vi "Ch_setup_string.vi"(6 "Ch & spans":T1[](array[typedef]) {"Sync Delay (ms)" format="%.3f"}) -> (1 "Output string":string)   [LabVIEW 2017]
uses:
  Controls/Ch_and_Spans.ctl
  Globals/Meas_global.vi
panel:
  out "length":i32
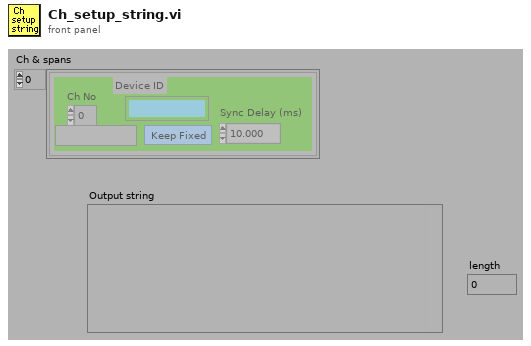
[diagram p1: front panel]
types:
  T1 = typedef "Ch_and_Spans.ctl" = cluster{"Sync Delay (ms)":dbl, "Ch No":i16, "Var name":string, "Use Latest Calib":bool, "Device ID":string}
  T2 = typedef "Analysis_info_cluster.ctl" = cluster{"Colour":u32, "Inst type":T3, "Inst name":string, "Symbol":string, "Code name":string, "Extra Info":string, "Inst Array":T4, "Extra Titles":string[], "Extra Values":string[], "U":dbl, "u^2":dbl, "u^3":dbl, "u^4":dbl, "Skew_u":dbl, "Kurt_u":dbl, "Sd Error in Mean":dbl, "% u'/U":dbl, "X":dbl, "Y":dbl, "Z":dbl, "Timescale integral Estimate":dbl, "Sd Error in Variance":dbl, "Calib File":path, "Calib Constants":dbl[], "Output Position":bool, "Full Stats":bool, "Av Sampling Rate":dbl, "Av No of Samples":dbl, "Total Meas Time (s)":dbl, "ADAM Ch Name":string, "Max value":dbl, "Min value":dbl, "Sync Delay Time (s)":dbl, "Device ID":string}
  T3 = typedef "Inst_type.ctl" = enum16{"Propeller anemometer", "Raw voltage", "Pressure Transducer", "Pitot-static tube", "Preston tube", "Hot wire", "Cross wire 1", "Cross wire 2", "Generic Linear", "Generic Polynomial", "Generic BackPoly", "Fast FID", "Thermocouple", "Cold wire", "Pulsed Wire", "LDA Vel", "LDA Tran time", "LDA Arr time", "Microphone"}
  T4 = typedef "Instrument_Array.ctl" = enum16{"PWA", "LDA", "Analogue"}
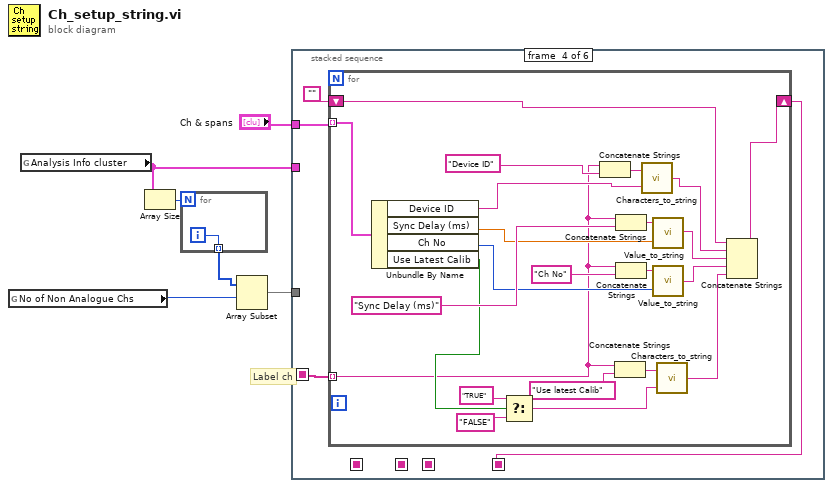
[diagram p0: block diagram]
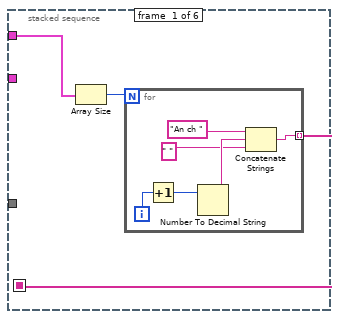
[diagram p2: hidden frame]
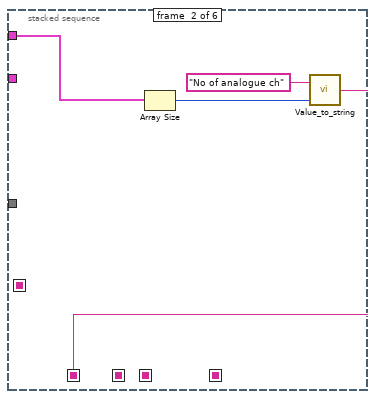
[diagram p3: hidden frame]
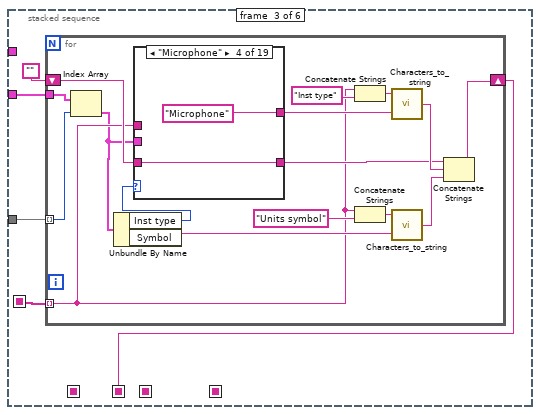
[diagram p4: hidden frame]
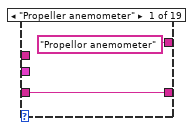
[diagram p5: hidden frame]
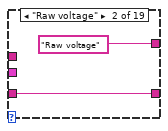
[diagram p6: hidden frame]
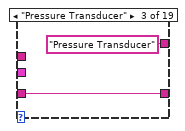
[diagram p7: hidden frame]
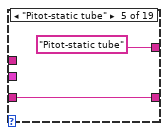
[diagram p8: hidden frame]
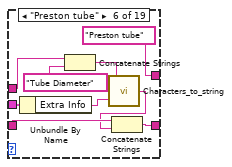
[diagram p9: hidden frame]
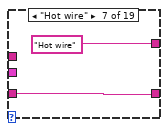
[diagram p10: hidden frame]
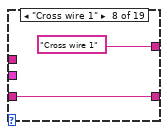
[diagram p11: hidden frame]
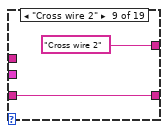
[diagram p12: hidden frame]
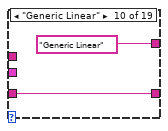
[diagram p13: hidden frame]
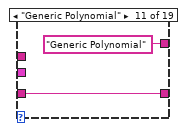
[diagram p14: hidden frame]
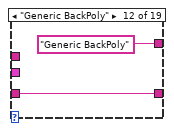
[diagram p15: hidden frame]
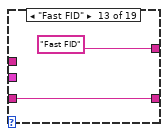
[diagram p16: hidden frame]
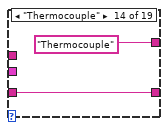
[diagram p17: hidden frame]
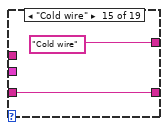
[diagram p18: hidden frame]
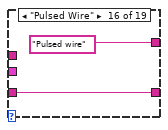
[diagram p19: hidden frame]
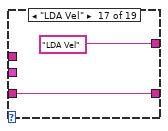
[diagram p20: hidden frame]
diagram:
  # "Label ch"
  n1 = global read "Meas_global.vi" "No of Non Analogue Chs"() -> (w2:i32)
  n2 = global read "Meas_global.vi" "Analysis Info cluster"() -> (w5:T2[])
  n3 = Array Size(array=w5) -> (size(s)=w4:i32)
  n4 = for {
    N: w4 -> [_]
    tunnel: [w7] -> w3 mode=indexing
    i -> [w7]
  }
  n5 = Array Subset(array=w3, index=w2) -> (w1:i32[])  [unwired: 1 in]
  n6 = stacked-sequence {
    seq-local: [_ _ w24 _ _ _] -> [_ _ _ _ _ w135]
    seq-local: [_ _ _ _ w116 _] -> [_ _ _ _ _ w134]
    seq-local: [w9 _ _ _ _ _] -> [_ _ w23 w89 w117 _]
    seq-local: [_ w17 _ _ _ _] -> [_ _ _ _ _ w131]
    seq-local: [_ _ _ w88 _ _] -> [_ _ _ _ _ w130]
    tunnel: "Ch & spans" -> [w8 w18 _ w87 _ _]
    tunnel: w5 -> [_ _ w22 _ w115 _]
    tunnel: w1 -> [_ _ w21 _ w114 _]
    frame #0 {
      n7 = Array Size(array=w8) -> (size(s)=w10:i32)
      n8 = for {
        N: w10 -> [_]
        tunnel: [w12] -> w9 mode=indexing
        i -> [w14]
        n9 = Increment(x=w14) -> (x+1=w13:i32)
        n10 = Number To Decimal String(number=w13) -> (decimal integer string=w16:string)  [unwired: 1 out]
        n11 = Concatenate Strings("An ch ", w16, " ") -> (w12:string)
      }
    }
    frame #1 {
      n12 = Array Size(array=w18) -> (size(s)=w19:i32)
      n13 = call "Value_to_string.vi"("Value"=w19, "Label for value"="No of analogue ch") -> ("Output string"=w17:string)  [unwired: 1 in]
    }
    frame #2 {
      n14 = for {
        shift-right: [w41] -> w24
        shift-left: "" -> [w32]
        tunnel: w23 -> [w29] mode=indexing
        tunnel: w22 -> [w28]
        tunnel: w21 -> [w27] mode=indexing
        n15 = Index Array(array=w28, index=w27) -> (element=w26:T2)
        n16 = Unbundle By Name(w26) -> ("Inst type"=w30:T3, "Symbol"=w40:string)
        n17 = case shown="\"Microphone\"" w30 {
          tunnel: ["Propellor anemometer" "Raw voltage" "Pressure Transducer" "Microphone" "Pitot-static tube" "Preston tube" "Hot wire" "Cross wire 1" "Cross wire 2" "Generic Linear" "Generic Polynomial" "Generic BackPoly" "Fast FID" "Thermocouple" "Cold wire" "Pulsed wire" "LDA Vel" "LDA Tran time" "LDA Arr time"] -> w39
          tunnel: w32 -> [w42 w44 w46 w48 w50 w58 w61 w63 w65 w67 w69 w71 w73 w75 w77 w79 w81 w83 w85]
          tunnel: [w42 w44 w46 w48 w50 w57 w61 w63 w65 w67 w69 w71 w73 w75 w77 w79 w81 w83 w85] -> w31
          tunnel: w26 -> [_ _ _ _ _ w60 _ _ _ _ _ _ _ _ _ _ _ _ _]
          tunnel: w29 -> [_ _ _ _ _ w53 _ _ _ _ _ _ _ _ _ _ _ _ _]
          frame "Propeller anemometer" {
          }
          frame "Raw voltage" {
          }
          frame "Pressure Transducer" {
          }
          frame "Microphone" {
          }
          frame "Pitot-static tube" {
          }
          frame "Preston tube" {
            n18 = Unbundle By Name(w60) -> ("Extra Info"=w59:string)
            n19 = Concatenate Strings(w53, "Tube Diameter") -> (w52:string)
            n20 = call "Characters_to_string.vi"("Characters to write"=w59, "Label for characters"=w52) -> ("Output string"=w55:string)
            n21 = Concatenate Strings(w58, w55) -> (w57:string)
          }
          frame "Hot wire" {
          }
          frame "Cross wire 1" {
          }
          frame "Cross wire 2" {
          }
          frame "Generic Linear" {
          }
          frame "Generic Polynomial" {
          }
          frame "Generic BackPoly" {
          }
          frame "Fast FID" {
          }
          frame "Thermocouple" {
          }
          frame "Cold wire" {
          }
          frame "Pulsed Wire" {
          }
          frame "LDA Vel" {
          }
          frame "LDA Tran time" {
          }
          frame "LDA Arr time" {
          }
        }
        n22 = Concatenate Strings(w29, "Inst type") -> (w33:string)
        n23 = Concatenate Strings(w29, "Units symbol") -> (w34:string)
        n24 = call "Characters_to_string.vi"("Characters to write"=w39, "Label for characters"=w33) -> ("Output string"=w35:string)
        n25 = call "Characters_to_string.vi"("Characters to write"=w40, "Label for characters"=w34) -> ("Output string"=w36:string)
        n26 = Concatenate Strings(w31, w35, w36) -> (w41:string)
      }
    }
    frame #3 {
      n27 = for {
        shift-right: [w113] -> w88
        shift-left: "" -> [w97]
        tunnel: w89 -> [w91] mode=indexing
        tunnel: w87 -> [w100] mode=indexing
        n28 = Unbundle By Name(w100) -> ("Device ID"=w94:string, "Sync Delay (ms)"=w106:dbl, "Ch No"=w107:i16, "Use Latest Calib"=w99:bool)
        n29 = Select(t="TRUE", s=w99, f="FALSE") -> (s? t:f=w101:string)
        n30 = Concatenate Strings(w91, "Device ID") -> (w96:string)
        n31 = Concatenate Strings(w91, "Use latest Calib") -> (w104:string)
        n32 = Concatenate Strings(w91, "Sync Delay (ms)") -> (w95:string)
        n33 = Concatenate Strings(w91, "Ch No") -> (w110:string)
        n34 = call "Characters_to_string.vi"("Characters to write"=w94, "Label for characters"=w96) -> ("Output string"=w93:string)
        n35 = call "Value_to_string.vi"("Value"=w106, "Label for value"=w95) -> ("Output string"=w109:string)  [unwired: 1 in]
        n36 = call "Value_to_string.vi"("Value"=w107, "Label for value"=w110) -> ("Output string"=w108:string)  [unwired: 1 in]
        n37 = call "Characters_to_string.vi"("Characters to write"=w101, "Label for characters"=w104) -> ("Output string"=w98:string)
        n38 = Concatenate Strings(w97, w93, w109, w108, w98) -> (w113:string)
      }
    }
    frame #4 {
      n39 = for {
        shift-right: [w128] -> w116
        shift-left: "" -> [w129]
        tunnel: w117 -> [w124] mode=indexing
        tunnel: w115 -> [w121]
        tunnel: w114 -> [w120] mode=indexing
        n40 = Index Array(array=w121, index=w120) -> (element=w119:T2)
        n41 = Unbundle By Name(w119) -> ("Calib File"=w122:path)
        n42 = Path To String(path=w122) -> (string=w123:string)
        n43 = Concatenate Strings(w124, "Calib filename") -> (w125:string)
        n44 = call "Characters_to_string.vi"("Characters to write"=w123, "Label for characters"=w125) -> ("Output string"=w126:string)
        n45 = Concatenate Strings(w129, w126) -> (w128:string)
      }
    }
    frame #5 {
      n46 = Concatenate Strings(w131, w135, w134, w130) -> (w132:string)
      "Output string" <- w132
      n47 = String Length(string=w132) -> (length=→"length":i32)
    }
  }
